vi "Write trusted entities.vi"(8 "error in (no error)":errorcluster, 10 "trusted entities":path[](array[path]), 11 "Connection.TCP-TLS in":refnum<class "Connection.TCP-TLS.lvclass">) -> (0 "error out":errorcluster, 3 "Connection.TCP-TLS out":refnum<class "Connection.TCP-TLS.lvclass">)   [LabVIEW 2020, in "Connection.TCP-TLS.lvclass"]
uses:
  Connection.TCP-TLS.lvclass
  Connection.TCP-TLS.lvclass/Connection.TCP-TLS.ctl
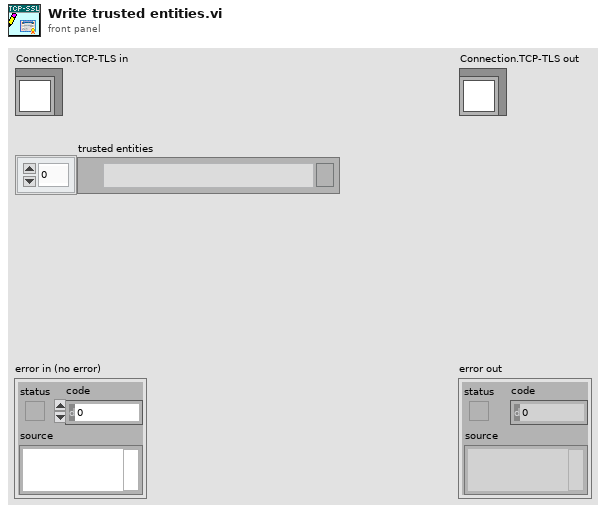
[diagram p1: front panel]
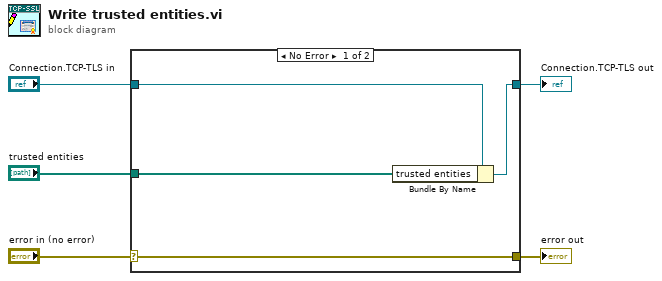
[diagram p0: block diagram]
diagram:
  n1 = case shown="No Error" "error in (no error)" {
    selector: "error in (no error)" -> [w9 w10]
    tunnel: [w9 w10] -> w4
    tunnel: [w7 w11] -> w2
    tunnel: "Connection.TCP-TLS in" -> [w8 w11]
    tunnel: "trusted entities" -> [w6 _]
    frame No Error {
      n2 = Bundle By Name(cluster=w8, "trusted entities"=w6) -> (w7:refnum<class "Connection.TCP-TLS.lvclass">)
    }
    frame Error {
    }
  }
  "error out" <- w4
  "Connection.TCP-TLS out" <- w2
